vi "Parse Comments and Commands.vi"(3 "ITX Notes and Commands":string) -> (0 "Commands":string, 1 "Notes":string)   [LabVIEW 2019, in "LV-Data.ITX.lvclass"]
uses:
  LV-Data.ITX.lvclass
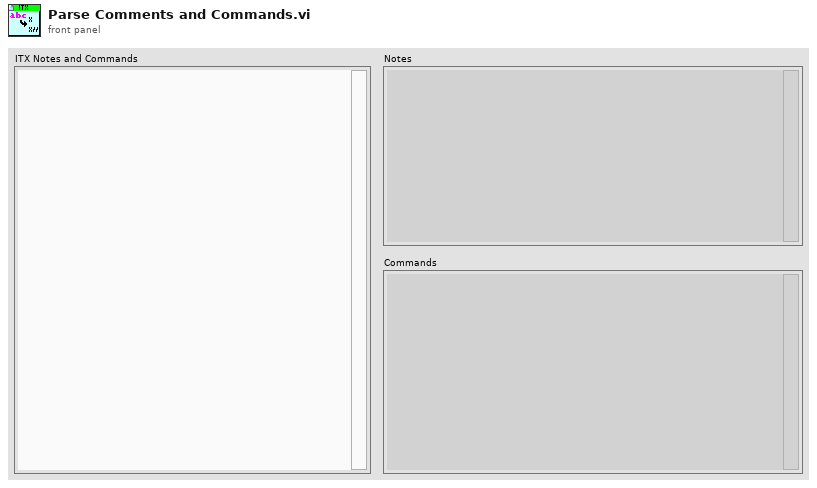
[diagram p1: front panel]
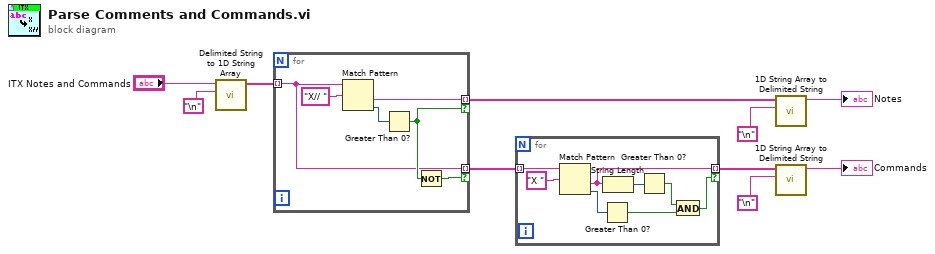
[diagram p0: block diagram]
diagram:
  n1 = call <vilib>:"Delimited String to 1D String Array.vi"("delimiter"="\n", "delimited string"="ITX Notes and Commands") -> ("string array"=w7:string[])  [unwired: 9 in]
  n2 = for {
    tunnel: w7 -> [w11] mode=indexing
    tunnel: [w14] -> w5 mode=indexing if=w12
    tunnel: [w11] -> w10 mode=indexing if=w16
    n3 = Match Pattern(string=w11, regular expression="X// " ("String")) -> (after substring=w14:string, offset past match=w13:i32)  [unwired: 3 out]
    n4 = Greater Than 0?(x=w13) -> (x > 0?=w12:bool)
    n5 = Not(x=w12) -> (.not. x?=w16:bool)
  }
  n6 = for {
    tunnel: w10 -> [w23] mode=indexing
    tunnel: [w21] -> w3 mode=indexing if=w17
    n7 = Match Pattern(string=w23, regular expression="X " ("String")) -> (after substring=w21:string, offset past match=w22:i32)  [unwired: 3 out]
    n8 = Greater Than 0?(x=w22) -> (x > 0?=w18:bool)
    n9 = String Length(string=w21) -> (length=w20:i32)
    n10 = Greater Than 0?(x=w20) -> (x > 0?=w19:bool)
    n11 = And(x=w19, y=w18) -> (x .and. y?=w17:bool)
  }
  n12 = call <vilib>:"1D String Array to Delimited String.vi"("delimiter"="\n", "string array"=w5) -> ("delimited string"=→"Notes":string)  [unwired: 9 in]
  n13 = call <vilib>:"1D String Array to Delimited String.vi"("delimiter"="\n", "string array"=w3) -> ("delimited string"=→"Commands":string)  [unwired: 9 in]
